vi "Initialize.vi"(5 "components directory":path, 7 "options":T1, 8 "error in (no error)":errorcluster, 10 "framework configuration":T6, 11 "Framework in":refnum<class "Framework.lvclass">) -> (0 "error out":errorcluster, 3 "Framework out":refnum<class "Framework.lvclass">)   [LabVIEW 2017, in "DSF Core.lvlib" / "Framework.lvclass"]
uses:
  Framework.lvclass
  Typedefs/DSF Engine Framework Configuration.ctl
  Typedefs/DSF Engine Plugin Configuration.ctl
  Typedefs/DSF Timing Info.ctl
  Typedefs/DSF Engine Plugin Thread Configuration.ctl
  Typedefs/DSF Settings Info.ctl
  Typedefs/DSF Engine Transfer Group Configuration.ctl
  Typedefs/DSF Direction.ctl
  Typedefs/DSF Engine Transfer Configuration.ctl
  Typedefs/DSF Byte Order.ctl
  Typedefs/DSF Engine Channel Configuration.ctl
  Typedefs/DSF Data Type.ctl
  Typedefs/DSF Timeout Behavior.ctl
  Framework Options.ctl
  Typedefs/DSF FIFO Options.ctl
  Thread/DSF Thread Options.ctl
  Typedefs/DSF Plugin Options.ctl
  Typedefs/DSF Performance Options.ctl
  Framework.lvclass/Framework.ctl
  Dispatcher/Dispatcher Thread.lvclass
  C:/Git/DSF/Data Sharing Framework/Source/Core/Classes/Thread/Thread.lvclass
  Thread/Plugin/Plugin Thread.lvclass
  Thread Manager/Thread Manager.lvclass
  Performance/Performance.lvclass
  DSF Core.lvlib
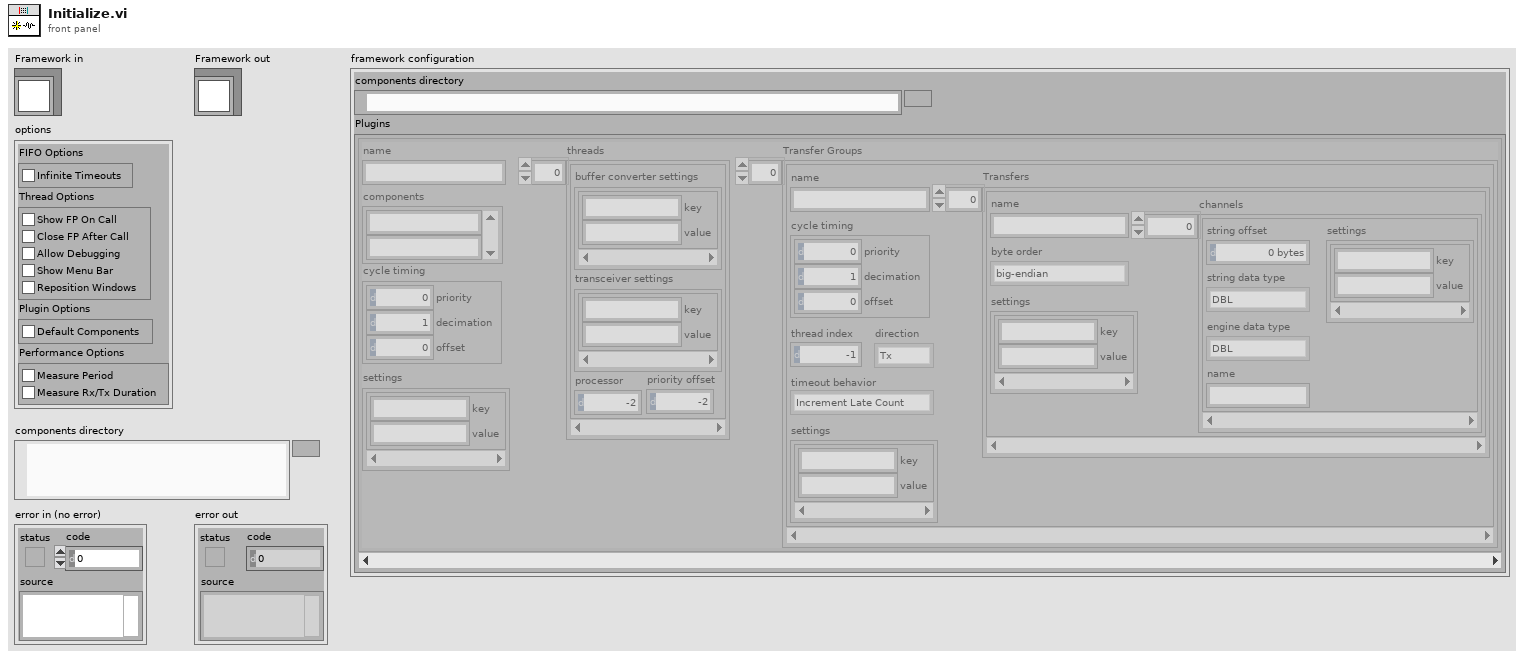
[diagram p1: front panel]
types:
  T1 = typedef "DSF Core.lvlib/Framework.lvclass/Framework Options.ctl" = cluster{"FIFO Options":T2, "Thread Options":T3, "Plugin Options":T4, "Performance Options":T5}
  T2 = typedef "DSF Core.lvlib/DSF FIFO Options.ctl" = cluster{"Infinite Timeouts":bool}
  T3 = typedef "DSF Core.lvlib/DSF Thread Options.ctl" = cluster{"Show FP On Call":bool, "Close FP After Call":bool, "Allow Debugging":bool, "Show Menu Bar":bool, "Reposition Windows":bool}
  T4 = typedef "DSF Core.lvlib/DSF Plugin Options.ctl" = cluster{"Default Components":bool}
  T5 = typedef "DSF Core.lvlib/DSF Performance Options.ctl" = cluster{"Measure Period":bool, "Measure Rx/Tx Duration":bool}
  T6 = typedef "DSF Core.lvlib/DSF Engine Framework Configuration.ctl" = cluster{"components directory":path, "Plugins":T7[]}
  T7 = typedef "DSF Core.lvlib/DSF Engine Plugin Configuration.ctl" = cluster{"name":string, "components":string[], "cycle timing":T8, "threads":T9[], "Transfer Groups":T11[], "settings":T10}
  T8 = typedef "DSF Core.lvlib/DSF Timing Info.ctl" = cluster{"priority":u64, "decimation":u64, "offset":u64}
  T9 = typedef "DSF Core.lvlib/DSF Engine Plugin Thread Configuration.ctl" = cluster{"buffer converter settings":T10, "transceiver settings":T10, "processor":i32, "priority offset":i16}
  T10 = typedef "DSF Core.lvlib/DSF Settings Info.ctl" = cluster{"key":string, "value":string}[]
  T11 = typedef "DSF Core.lvlib/DSF Engine Transfer Group Configuration.ctl" = cluster{"name":string, "direction":T12, "cycle timing":T8, "thread index":i32, "settings":T10, "Transfers":T13[], "timeout behavior":T17}
  T12 = typedef "DSF Core.lvlib/DSF Direction.ctl" = enum8{"Tx", "Rx"}
  T13 = typedef "DSF Core.lvlib/DSF Engine Transfer Configuration.ctl" = cluster{"name":string, "byte order":T14, "settings":T10, "channels":T15[]}
  T14 = typedef "DSF Core.lvlib/DSF Byte Order.ctl" = enum8{"big-endian", "little-endian"}
  T15 = typedef "DSF Core.lvlib/DSF Engine Channel Configuration.ctl" = cluster{"string offset":u64, "string data type":T16, "engine data type":T16, "name":string, "settings":T10}
  T16 = typedef "DSF Core.lvlib/DSF Data Type.ctl" = enum8{"Bool", "SGL", "DBL", "I8", "I16", "I32", "I64", "U8", "U16", "U32", "U64"}
  T17 = typedef "DSF Core.lvlib/DSF Timeout Behavior.ctl" = enum8{"Increment Late Count", "Throw Error"}
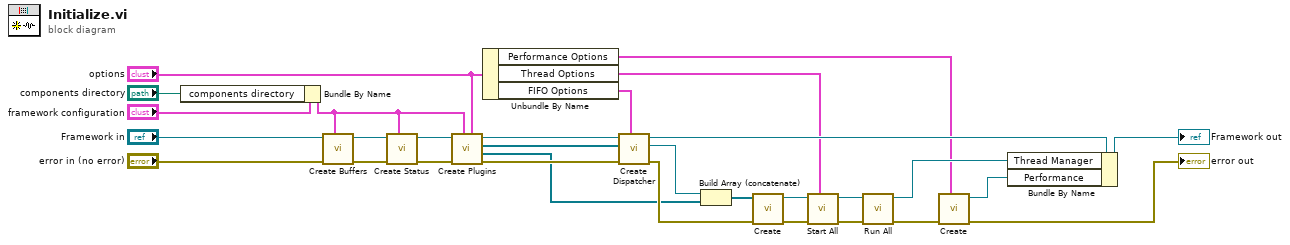
[diagram p0: block diagram]
diagram:
  n1 = Bundle By Name(cluster="framework configuration", "components directory"="components directory") -> (w7:T6)
  n2 = call "Create Buffers.vi"("framework configuration"=w7, "error in (no error)"="error in (no error)", "Framework in"="Framework in") -> ("error out"=w5:errorcluster, "Framework out"=w6:refnum<class "Framework.lvclass">)  [unwired: 7 in]
  n3 = call "Create Status.vi"("Framework Configuration"=w7, "error in (no error)"=w5, "Framework in"=w6) -> ("error out"=w3:errorcluster, "Framework out"=w4:refnum<class "Framework.lvclass">)  [unwired: 7 in]
  n4 = call "Create Plugins.vi"("options"="options", "framework configuration"=w7, "error in (no error)"=w3, "Framework in"=w4) -> ("error out"=w29:errorcluster, "Plugin Threads"=w8:refnum<class "Plugin Thread.lvclass">[], "Plugins"=w18:refnum<class "Plugin.lvclass">[], "Framework out"=w30:refnum<class "Framework.lvclass">)  [unwired: 4 in]
  n5 = Unbundle By Name("options") -> ("Performance Options"=w11:T5, "Thread Options"=w17:T3, "FIFO Options"=w16:T2)
  n6 = call "Create Dispatcher.vi"("FIFO Options"=w16, "error in (no error)"=w29, "Plugins"=w18, "Framework in"=w30) -> ("error out"=w25:errorcluster, "Dispatcher Thread"=w9:refnum<class "Dispatcher Thread.lvclass">, "Framework out"=w26:refnum<class "Framework.lvclass">)  [unwired: 5 in]
  n7 = Build Array (concatenate)(w9, w8) -> (w10:refnum<class "Thread.lvclass">[])
  n8 = call "Create.vi"("error in (no error)"=w25, "Threads"=w10) -> ("error out"=w23:errorcluster, "Thread Manager"=w24:refnum<class "Thread Manager.lvclass">)  [unwired: 8 in]
  n9 = call "Start All.vi"("options"=w17, "error in (no error)"=w23, "Thread Manager in"=w24) -> ("error out"=w21:errorcluster, "Thread Manager out"=w22:refnum<class "Thread Manager.lvclass">)  [unwired: 7 in]
  n10 = call "Run All.vi"("error in (no error)"=w21, "Thread Manager in"=w22) -> ("error out"=w13:errorcluster, "Thread Manager out"=w20:refnum<class "Thread Manager.lvclass">)  [unwired: 8 in]
  n11 = call "Create.vi"("options (all enabled)"=w11, "error in (no error)"=w13) -> ("error out"=→"error out":errorcluster, "performance"=w12:refnum<class "Performance.lvclass">)  [unwired: 8 in]
  n12 = Bundle By Name(cluster=w26, "Thread Manager"=w20, "Performance"=w12) -> (→"Framework out":refnum<class "Framework.lvclass">)
